vi "GNSS RF Test Get Default Parameters.vi"(8 "error in (no error)":errorcluster, 11 "Template Tx Test in":refnum<class "niDTS GNSS RF Test.lvclass">) -> (0 "error out":errorcluster, 2 "Parameters":T1={"GNSS Standard"=enum."GPS", "Frequency (Hz)"=1575420000.0, "Auto Level"=FALSE, "Power (dBm)"=0.0, "External Attenuation (dB)"=0.0, "Measurement Interval (s)"=1.0, "Pattern"=enum."PN9", "Enable Averaging"=FALSE, "Type Of Averaging"=enum."MEAN", "Number of Averages"=1, "Waveform Name"="", "Enable Traces"=FALSE} {"External Attenuation (dB)" format="%.1g"; "Power (dBm)" format="%.1g"}, 3 "Template Tx Test out":refnum<class "niDTS GNSS RF Test.lvclass">)   [LabVIEW 2015, in "niDTS GNSS.lvlib" / "niDTS GNSS RF Test.lvclass"]
uses:
  niDTS GNSS RF Test.lvclass
  Includes/niDTS GNSS RF Test INC Parameters.ctl
  niDTS GNSS RF Test.lvclass/niDTS GNSS RF Test.ctl
  niDTS GNSS.lvlib
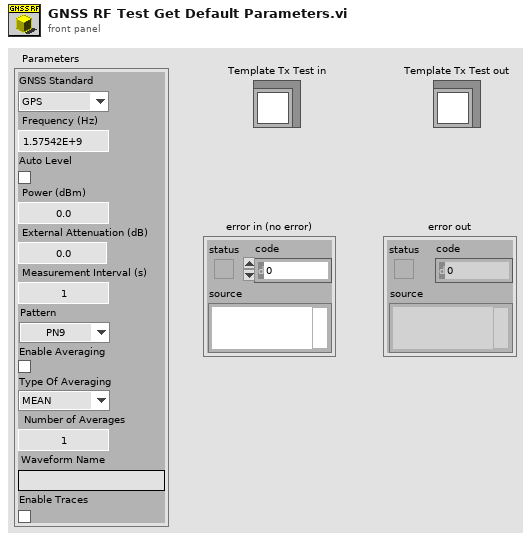
[diagram p1: front panel]
types:
  T1 = typedef "niDTS GNSS.lvlib/niDTS GNSS RF Test INC Parameters.ctl" = cluster{"GNSS Standard":enum16{"GPS", "GLONASS", "Galileo", "Beidou"}, "Frequency (Hz)":dbl, "Auto Level":bool, "Power (dBm)":dbl, "External Attenuation (dB)":dbl, "Measurement Interval (s)":dbl, "Pattern":enum16{"0", "1", "01", "00001111", "PN9"}, "Enable Averaging":bool, "Type Of Averaging":enum16{"MEAN", "MAX", "MIN", "MAXMIN"}, "Number of Averages":i32, "Waveform Name":string, "Enable Traces":bool}
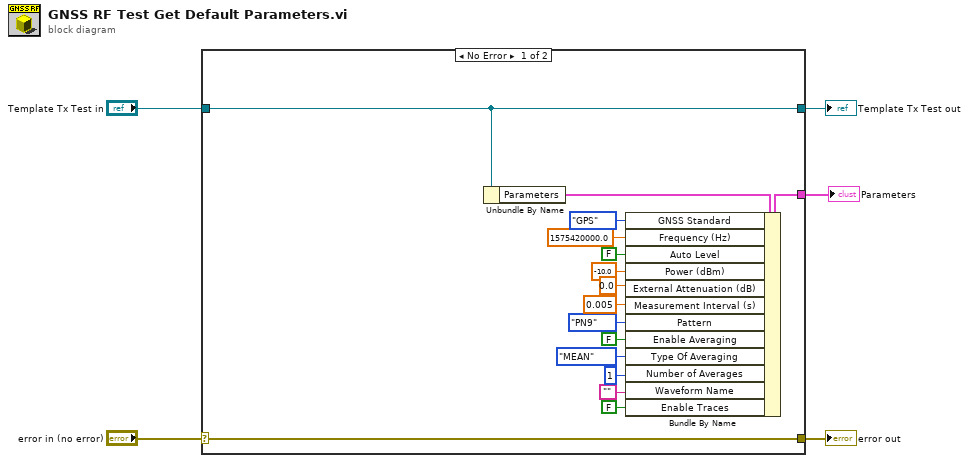
[diagram p0: block diagram]
diagram:
  n1 = case shown="No Error" "error in (no error)" {
    selector: "error in (no error)" -> [w21 w23]
    tunnel: [w21 w23] -> w4
    tunnel: [w20 w22] -> w2
    tunnel: "Template Tx Test in" -> [w20 w22]
    tunnel: [w18 _] -> w1
    frame No Error {
      n2 = Unbundle By Name(w20) -> ("Parameters"=w19:T1)
      n3 = Bundle By Name(cluster=w19, "GNSS Standard"=enum16{"GPS", "GLONASS", "Galileo", "Beidou"}."GPS", "Frequency (Hz)"=1575420000.0, "Auto Level"=FALSE, "Power (dBm)"=-10.0, "External Attenuation (dB)"=0.0, "Measurement Interval (s)"=0.005, "Pattern"=enum16{"0", "1", "01", "00001111", "PN9"}."PN9", "Enable Averaging"=FALSE, "Type Of Averaging"=enum16{"MEAN", "MAX", "MIN", "MAXMIN"}."MEAN", "Number of Averages"=1, "Waveform Name"="", "Enable Traces"=FALSE) -> (w18:T1)
    }
    frame Error {
    }
  }
  "error out" <- w4
  "Template Tx Test out" <- w2
  "Parameters" <- w1
